vi "ADIS16448_RoboRIO_Teensy_Reset.vi"(8 "error in":errorcluster, 11 "SerialPortRef":T1) -> (0 "error out":errorcluster, 3 "SerialPortRefOut":T1)   [LabVIEW 2016, in "RoboRIO-Teensy-ADIS16448-Interface.lvlib"]
uses:
  RoboRIO-Teensy-ADIS16448-Interface.lvlib
  <vilib>/Rock Robotics/WPI/SerialPort/WPI_SerialPortRef.ctl
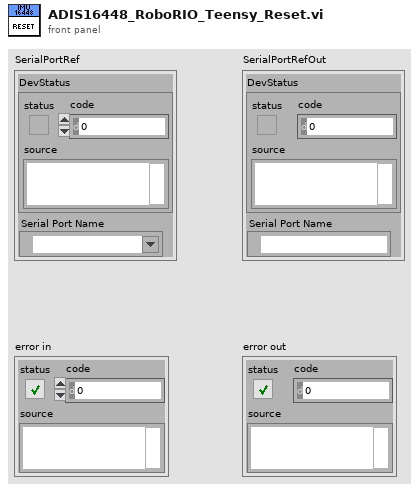
[diagram p1: front panel]
types:
  T1 = typedef "WPI_SerialPortRef.ctl" = cluster{"DevStatus":errorcluster, "Serial Port Name":refnum<visa-resource-name>}
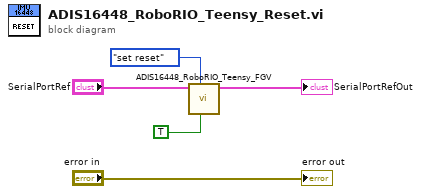
[diagram p0: block diagram]
diagram:
  n1 = call "ADIS16448_RoboRIO_Teensy_FGV.vi"("Reset"=TRUE, "Operation"=enum16{"set", "get", "set reset"}."set reset", "SerialPortRefIn"="SerialPortRef") -> ("SerialPortRefOut"=→"SerialPortRefOut":T1)  [unwired: 4 in, 4 out]
  "error out" <- "error in"
